vi "FL_Calculate_phi_theta_etc_2.vi"(0 "Input cluster of data":T1, 1 "SB size":u8, 2 "Bridge swap":bool, 3 "Use alternative magnets orientation":bool, 4 "Twisted neck":bool) -> (5 "Animal coordinates":T2)   [LabVIEW 2018, in "Tracker.lvlib"]
uses:
  Tracker.lvlib
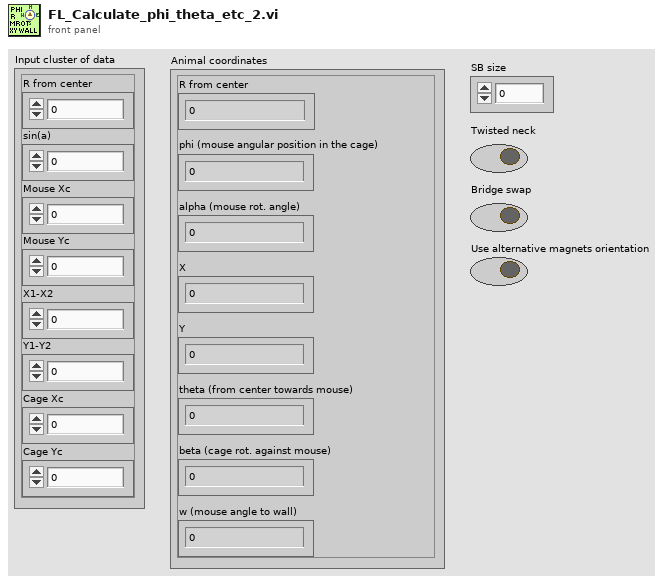
[diagram p1: front panel]
types:
  T1 = cluster{"R from center":dbl, "sin(a)":dbl, "Mouse Xc":dbl, "Mouse Yc":dbl, "X1-X2":dbl, "Y1-Y2":dbl, "Cage Xc":dbl, "Cage Yc":dbl}
  T2 = cluster{"R from center":dbl, "phi (mouse angular position in the cage)":dbl, "alpha (mouse rot. angle)":sgl, "X":dbl, "Y":dbl, "theta (from center towards mouse)":dbl, "beta (cage rot. against mouse)":sgl, "w (mouse angle to wall)":dbl}
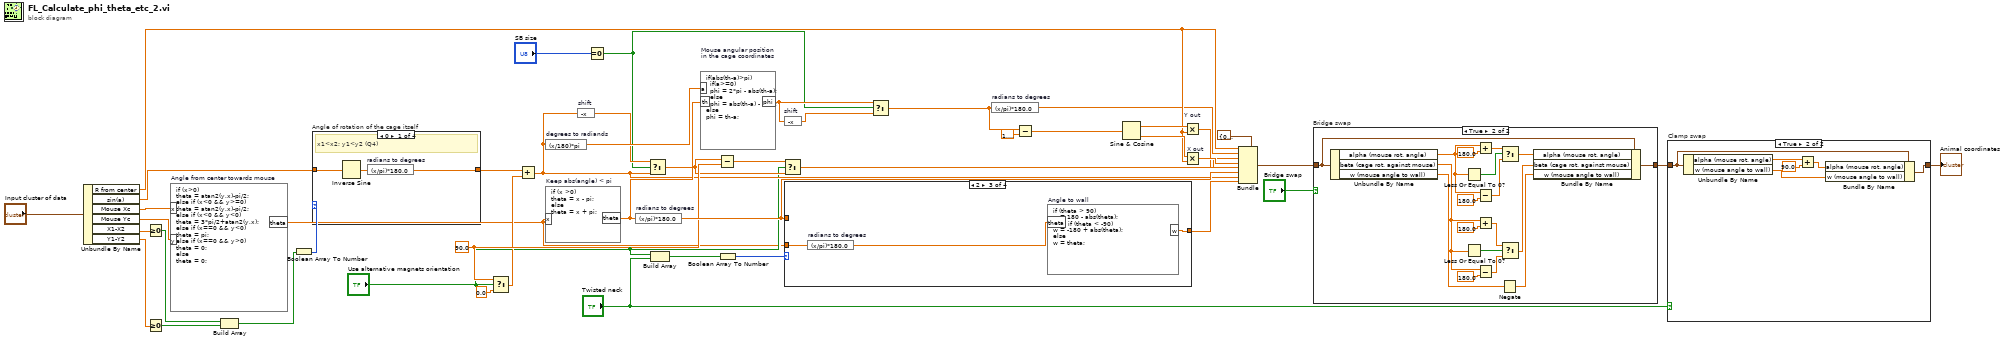
[diagram p0: block diagram]
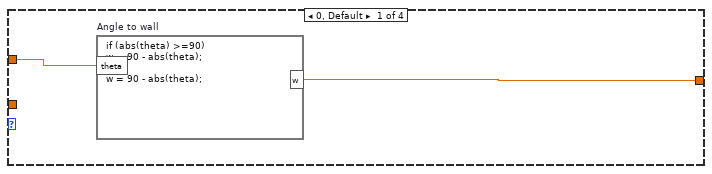
[diagram p3: hidden frame]
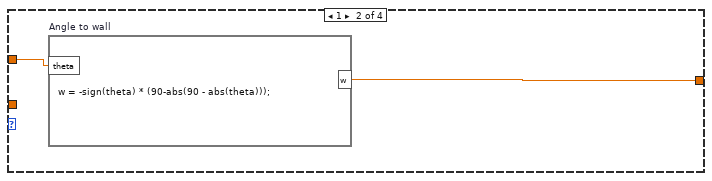
[diagram p4: hidden frame]
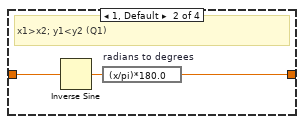
[diagram p7: hidden frame]
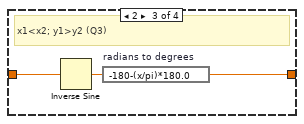
[diagram p8: hidden frame]
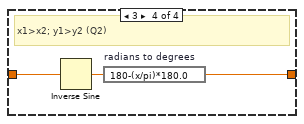
[diagram p9: hidden frame]
diagram:
  w18 = 90.0 ("y")
  n1 = Unbundle By Name("Input cluster of data") -> ("R from center"=w27:dbl, "sin(a)"=w32:dbl, "Mouse Xc"=w31:dbl, "Mouse Yc"=w30:dbl, "X1-X2"=w29:dbl, "Y1-Y2"=w28:dbl)
  n2 = Greater Or Equal To 0?(x=w29) -> (x >= 0?=w46:bool)
  n3 = Greater Or Equal To 0?(x=w28) -> (x >= 0?=w45:bool)
  n4 = formula code="if (x>0)\ntheta = atan2(y,x)-pi/2;\nelse if (x<0 && y>=0)\ntheta = atan2(y,x)-pi/2;\nelse if (x<0 && y<0)\ntheta = 3*pi/2+atan2(y,x);\nelse if (x==0 && y<0)\ntheta = pi;\nelse if (x==0 && y>0)\ntheta = 0;\nelse\ntheta = 0;" "Angle from center towards mouse"("x"=w31, "y"=w30) -> ("theta"=w3:dbl)
  n5 = Build Array(w46, w45) -> (w44:bool[])
  n6 = Boolean Array To Number(Boolean array=w44) -> (number=w43:u32)
  n7 = case "Angle of rotation of the cage itself" shown="0" w43 {
    tunnel: w32 -> [w48 w51 w54 w57]
    tunnel: [w47 w50 w53 w56] -> w21
    frame 0 {
      # "x1<x2; y1<y2 (Q4)"
      n8 = Inverse Sine(1:w48) -> (0:w49:dbl)
      n9 = expression code="(x/pi)*180.0" "radians to degrees"(w49) -> (w47:dbl)
    }
    frame 1, Default {
      # "x1>x2; y1<y2 (Q1)"
      n10 = Inverse Sine(1:w51) -> (0:w52:dbl)
      n11 = expression code="(x/pi)*180.0" "radians to degrees"(w52) -> (w50:dbl)
    }
    frame 2 {
      # "x1<x2; y1>y2 (Q3)"
      n12 = Inverse Sine(1:w54) -> (0:w55:dbl)
      n13 = expression code="-180-(x/pi)*180.0" "radians to degrees"(w55) -> (w53:dbl)
    }
    frame 3 {
      # "x1>x2; y1>y2 (Q2)"
      n14 = Inverse Sine(1:w57) -> (0:w58:dbl)
      n15 = expression code="180-(x/pi)*180.0" "radians to degrees"(w58) -> (w56:dbl)
    }
  }
  n16 = Select(t=w18, s="Use alternative magnets orientation", f=0.0) -> (s? t:f=w17:dbl)
  n17 = Add(x=w21, y=w17) -> (x+y=w15:dbl)
  n18 = expression code="(x/180)*pi" "degrees to radiands"(w15) -> (w39:dbl)
  n19 = formula code="if (x >0)\ntheta = x - pi;\nelse\ntheta = x + pi;" "Keep abs(angle) < pi"("x"=w3) -> ("theta"=w40:dbl)
  n20 = expression code="-x" "shift"(w15) -> (w14:dbl)
  n21 = Equal To 0?(x="SB size") -> (x = 0?=w1:bool)
  n22 = expression code="(x/pi)*180.0" "radians to degrees"(w40) -> (w34:dbl)
  n23 = Select(t=w14, s=w1, f=w15) -> (s? t:f=w16:dbl)
  n24 = Build Array("Use alternative magnets orientation", "Twisted neck") -> (w5:bool[])
  n25 = formula code="if(abs(th-a)>pi)\n  if(a>=0)\n  phi = 2*pi - abs(th-a);\n  else\n  phi = abs(th-a) - 2*pi;\nelse\nphi = th-a;" "Mouse angular position in the cage coordinates"("th"=w40, "a"=w39) -> ("phi"=w12:dbl)
  n26 = Subtract(x=w16, y=w18) -> (x-y=w19:dbl)
  n27 = Boolean Array To Number(Boolean array=w5) -> (number=w4:u32)
  n28 = Select(t=w19, s="Use alternative magnets orientation", f=w16) -> (s? t:f=w20:dbl)
  n29 = expression code="-x" "shift"(w12) -> (w11:dbl)
  n30 = case shown="2" w4 {
    tunnel: w34 -> [w60 w62 _ w66]
    tunnel: [w59 w61 w65 w66] -> w8
    tunnel: w3 -> [_ _ w64 _]
    frame 0, Default {
      n31 = formula code="if (abs(theta) >=90)\nw = 90 - abs(theta);\nelse\nw = 90 - abs(theta);" "Angle to wall"("theta"=w60) -> ("w"=w59:dbl)
    }
    frame 1 {
      n32 = formula code="w = -sign(theta) * (90-abs(90 - abs(theta)));" "Angle to wall"("theta"=w62) -> ("w"=w61:dbl)
    }
    frame 2 {
      n33 = expression code="(x/pi)*180.0" "radians to degrees"(w64) -> (w63:dbl)
      n34 = formula code="if (theta > 90)\nw = 180 - abs(theta);\nelse if (theta < -90)\nw = -180 + abs(theta);\nelse\nw = theta;" "Angle to wall"("theta"=w63) -> ("w"=w65:dbl)
    }
    frame 3 {
    }
  }
  n35 = Select(t=w12, s=w1, f=w11) -> (s? t:f=w13:dbl)
  n36 = expression code="(x/pi)*180.0" "radians to degrees"(w13) -> (w26:dbl)
  n37 = Subtract(x=w13, y=1.5707963267948966) -> (x-y=w38:dbl)
  n38 = Sine & Cosine(0:w38) -> (1:w41:dbl, 2:w42:dbl)
  n39 = Multiply "Y out"(x=w41, y=w27) -> (x*y=w35:dbl)
  n40 = Multiply "X out"(x=w42, y=w27) -> (x*y=w36:dbl)
  n41 = Bundle(cluster=T2 {"R from center"=0.0, "phi (mouse angular position in the cage)"=0.0, "alpha (mouse rot. angle)"=0.0, "X"=0.0, "Y"=0.0, "theta (from center towards mouse)"=0.0, "beta (cage rot. against mouse)"=0.0, "w (mouse angle to wall)"=0.0} ("Output data cluster 2"), "R from center"=w27, "phi (mouse angular position in the cage)"=w26, "alpha (mouse rot. angle)"=w20, "X"=w36, "Y"=w35, "theta (from center towards mouse)"=w34, "beta (cage rot. against mouse)"=w15, "w (mouse angle to wall)"=w8) -> (w23:T2)
  n42 = case "Bridge swap" shown="True" "Bridge swap" {
    tunnel: [w67 w79] -> w10
    tunnel: w23 -> [w67 w80]
    frame False {
    }
    frame True {
      n43 = Unbundle By Name(w80) -> ("alpha (mouse rot. angle)"=w78:sgl, "beta (cage rot. against mouse)"=w71:sgl, "w (mouse angle to wall)"=w69:dbl)
      n44 = Less Or Equal To 0?(x=w78) -> (x <= 0?=w85:bool)
      n45 = Less Or Equal To 0?(x=w71) -> (x <= 0?=w72:bool)
      n46 = Add(x=w78, y=sgl 180.0) -> (x+y=w82:sgl)
      n47 = Subtract(x=w78, y=sgl 180.0) -> (x-y=w84:sgl)
      n48 = Add(x=w71, y=sgl 180.0) -> (x+y=w75:sgl)
      n49 = Subtract(x=w71, y=sgl 180.0) -> (x-y=w73:sgl)
      n50 = Negate(x=w69) -> (-x=w68:dbl)
      n51 = Select(t=w82, s=w85, f=w84) -> (s? t:f=w77:sgl)
      n52 = Select(t=w75, s=w72, f=w73) -> (s? t:f=w70:sgl)
      n53 = Bundle By Name(cluster=w80, "alpha (mouse rot. angle)"=w77, "beta (cage rot. against mouse)"=w70, "w (mouse angle to wall)"=w68) -> (w79:T2)
    }
  }
  n54 = case "Clamp swap" shown="True" "Twisted neck" {
    tunnel: [w86 w90] -> w9
    tunnel: w10 -> [w86 w91]
    frame False {
    }
    frame True {
      n55 = Unbundle By Name(w91) -> ("alpha (mouse rot. angle)"=w89:sgl, "w (mouse angle to wall)"=w88:dbl)
      n56 = Add(x=w89, y=sgl 90.0) -> (x+y=w87:sgl)
      n57 = Bundle By Name(cluster=w91, "alpha (mouse rot. angle)"=w87, "w (mouse angle to wall)"=w88) -> (w90:T2)
    }
  }
  "Animal coordinates" <- w9
